vi "WPI_DriverStationStartStopVI.vi"(9 "VI in":refnum<vi>, 11 "Call Context":T1) -> ()   [LabVIEW 2017]
uses:
  <vilib>/Rock Robotics/WPI/DriverStation/WPI_DriverStationDerivedRobotMode.ctl
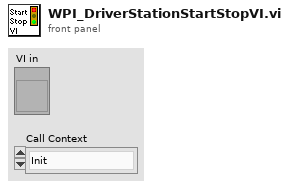
[diagram p1: front panel]
types:
  T1 = typedef "WPI_DriverStationDerivedRobotMode.ctl" = enum16{"Init", "Execute", "Stop"}
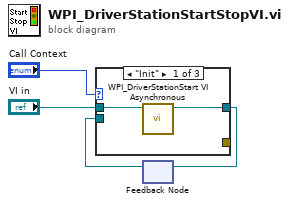
[diagram p0: block diagram]
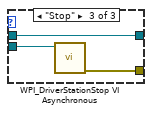
[diagram p3: hidden frame]
diagram:
  n1 = feedback #1() -> (w3:refnum<vi>)  [unwired: 1 out]
  n2 = case shown="\"Init\"" "Call Context" {
    tunnel: "VI in" -> [w6 _ w9]
    tunnel: [w5 w7 w9] -> w2
    tunnel: w3 -> [_ w7 w10]
    tunnel: [_ _ w8] -> _
    frame "Init" {
      n3 = call <vilib>:"WPI_DriverStationStart VI Asynchronous.vi"("VI"=w6) -> ("VI out"=w5:refnum<vi>)  [unwired: 10 out]
    }
    frame "Execute", Default {
      # "Running in parallel"
    }
    frame "Stop" {
      n4 = call <vilib>:"WPI_DriverStationStop VI Asynchronous.vi"("VI Refnum"=w10) -> ("error out"=w8:errorcluster)  [unwired: 10 out]
    }
  }
  n5 = feedback-in #1(w2) -> ()
